vi "Read.vi"(8 "error in (no error)":errorcluster, 11 "Local Bus_DBL":refnum<class "Fault-Injection_Variant.lvclass">) -> (0 "error out":errorcluster, 2 "Value":T1=variant(cdb 0.0+0.0i), 3 "Local Bus_DBL out":refnum<class "Fault-Injection_Variant.lvclass">)   [LabVIEW 2021, in "Fault-Injection_Variant.lvclass"]
uses:
  Fault-Injection_Variant.lvclass
  Support/Value Type.ctl
  Fault-Injection_Variant.lvclass/Fault-Injection_Variant.ctl
  <vilib>/TSA/Abstract Data Classes/Abs_Types/Variant/Abs_Variant.lvclass
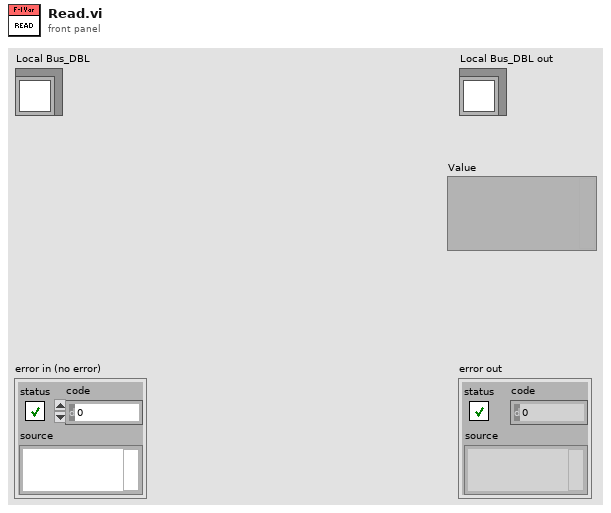
[diagram p1: front panel]
types:
  T1 = typedef "Fault-Injection_Variant.lvclass/Value Type.ctl" = variant
  T2 = typedef "Fault-Injection_Variant.lvclass/DVR Type.ctl" = cluster{"Enable":bool, "Injected Value":T1, "Value":T3}
  T3 = typedef "Fault-Injection_Variant.lvclass/Abs Class Type.ctl" = refnum<class "Abs_Variant.lvclass">
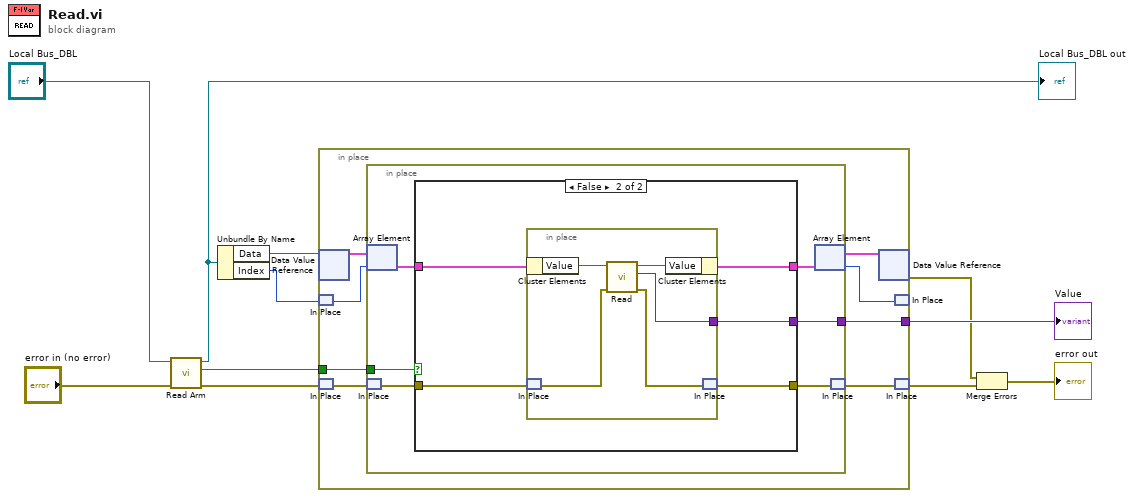
[diagram p0: block diagram]
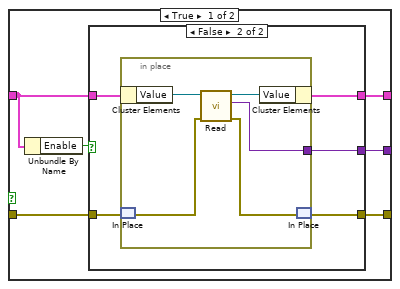
[diagram p2: hidden frame]
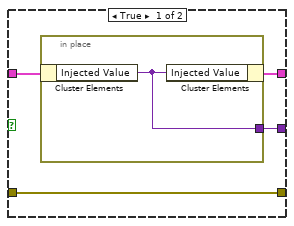
[diagram p3: hidden frame]
diagram:
  n1 = call "Read Arm.vi"("error in (no error)"="error in (no error)", "Fault-Injection_Boolean in"="Local Bus_DBL") -> ("error out"=w4:errorcluster, "Armed?"=w1:bool, "Fault-Injection_Boolean out"=w2:refnum<class "Fault-Injection_Variant.lvclass">)  [unwired: 7 in]
  "Local Bus_DBL out" <- w2
  n2 = Unbundle By Name(w2) -> ("Data"=w9:refnum<data-value>, "Index"=w8:i32)
  n3 = in-place {
    in-place-border: [w15] -> w11
    in-place-border: w1 -> [w12]
    n4 = in-place-dvr #1(w9) -> (w19:T2[])  [unwired: 1 out]
    n5 = in-place-match #2(w8) -> (w17:i32)
    n6 = in-place-match #3(w4) -> (w14:errorcluster)
    n7 = in-place {
      in-place-border: [w24] -> w15
      in-place-border: w12 -> [w20]
      n8 = in-place-array #4(w19, w17) -> (w21:T2)
      n9 = in-place-match #5(w14) -> (w23:errorcluster)
      n10 = case shown="False" w20 {
        tunnel: [w31 w51] -> w25
        tunnel: [w30 w50] -> w24
        tunnel: w23 -> [w29 w49]
        tunnel: [w28 w48] -> w22
        tunnel: w21 -> [w26 w47]
        frame True {
          n11 = Unbundle By Name(w26) -> ("Enable"=w27:bool)
          n12 = case shown="False" w27 {
            tunnel: w26 -> [w35 w41]
            tunnel: [w34 w40] -> w31
            tunnel: [w33 w39] -> w30
            tunnel: w29 -> [w32 w38]
            tunnel: [w32 w37] -> w28
            frame True {
              n13 = in-place {
                in-place-border: [w36] -> w33
                n14 = in-place-cluster #6(w35) -> ("Injected Value"=w36:T1)
                n15 = in-place-cluster #6("Injected Value"=w36) -> (w34:T2)
              }
            }
            frame False {
              n16 = in-place {
                in-place-border: [w42] -> w39
                n17 = in-place-cluster #7(w41) -> ("Value"=w43:T3)
                n18 = in-place-match #8(w38) -> (w45:errorcluster)
                n19 = call-dynamic "Read.vi"("error in (no error)"=w45, "Abs_Variant in"=w43) -> ("error out"=w44:errorcluster, "Variant"=w42:variant, "Abs_Variant out"=w46:T3)  [unwired: 7 in]
                n20 = in-place-cluster #7("Value"=w46) -> (w40:T2)
                n21 = in-place-match #8(w44) -> (w37:errorcluster)
              }
            }
          }
        }
        frame False {
          n22 = in-place {
            in-place-border: [w55] -> w50
            n23 = in-place-cluster #9(w47) -> ("Value"=w54:T3)
            n24 = in-place-match #10(w49) -> (w53:errorcluster)
            n25 = call-dynamic "Read.vi"("error in (no error)"=w53, "Abs_Variant in"=w54) -> ("error out"=w52:errorcluster, "Variant"=w55:variant, "Abs_Variant out"=w56:T3)  [unwired: 7 in]
            n26 = in-place-cluster #9("Value"=w56) -> (w51:T2)
            n27 = in-place-match #10(w52) -> (w48:errorcluster)
          }
        }
      }
      n28 = in-place-array #4(w25) -> (w18:T2[], w16:i32)
      n29 = in-place-match #5(w22) -> (w13:errorcluster)
    }
    n30 = in-place-dvr #1(w18) -> (w6:errorcluster)  [unwired: 1 out]
    n31 = in-place-match #2(w16) -> ()  [unwired: 1 out]
    n32 = in-place-match #3(w13) -> (w7:errorcluster)
  }
  "Value" <- w11
  n33 = Merge Errors(w6, w7) -> (→"error out":errorcluster)
